vi "IT6322_Config_Link.vi"(8 "error in":errorcluster caption="错误输入（无错误）", 10 "等待时间(毫秒)":u32=100, 11 "MyIndex":u8) -> (0 "error out":errorcluster, 2 "返回值":string, 3 "状态":bool)   [LabVIEW 2015, in "IT6322.lvlib"]
uses:
  IT6322.lvlib
  <vilib>/Instr/_visa.llb/VISA Configure Serial Port (Instr).vi
panel:
  out "VISA":refnum<visa-resource-name>
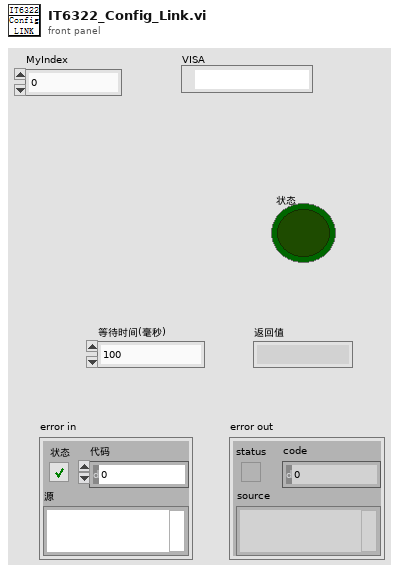
[diagram p1: front panel]
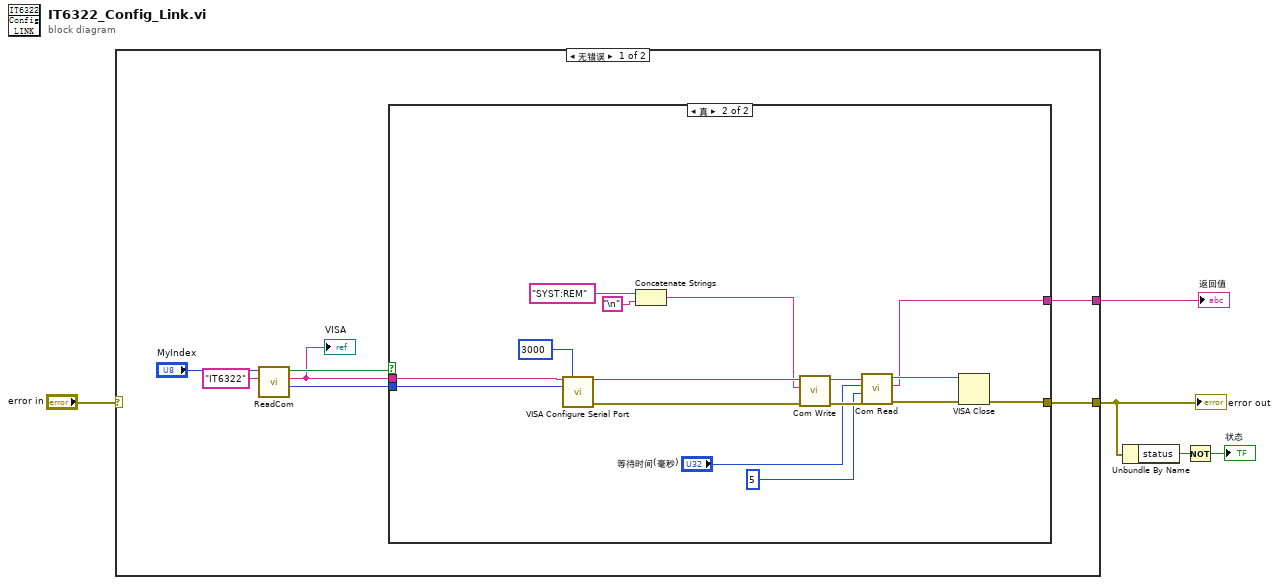
[diagram p0: block diagram]
diagram:
  n1 = case shown="无错误" "error in" {
    selector: "error in" -> [_ w29]
    tunnel: [w12 w29] -> w2
    tunnel: [w6 _] -> w3
    frame No Error {
      n2 = call "ReadCom.vi"("仪器名称"="IT6322", "MyIndex"="MyIndex") -> ("Baudrate"=w7:i32, "COM"=w8:string, "OK?"=w9:bool)  [unwired: 7 in]
      "VISA" <- w8
      n3 = case shown="真" w9 {
        tunnel: [_ w28] -> w12
        tunnel: w8 -> [_ w27]
        tunnel: w7 -> [_ w26]
        tunnel: [_ w18] -> w6
        frame False {
        }
        frame True {
          n4 = call-poly "VISA Configure Serial Port"("VISA resource name"=w27, "timeout (10sec)"=u32 3000, "baud rate (9600)"=w26) -> ("VISA resource name out"=w24:refnum<visa-resource-name>, "error out"=w23:errorcluster)  [unwired: 11 in]
          n5 = Concatenate Strings("SYST:REM", "\n") -> (w13:string)
          n6 = call "Com Write.vi"("错误输入（无错误）"=w23, "Wbuff"=w13, "VISA In"=w24) -> ("错误输出"=w21:errorcluster, "VISA Out"=w22:refnum<visa-resource-name>)  [unwired: 7 in]
          n7 = call "Com Read.vi"("错误输入（无错误）"=w21, "num"=u32 5, "超时"="等待时间(毫秒)", "VISA In"=w22) -> ("错误输出"=w20:errorcluster, "buff"=w18:string, "VISA Out"=w19:refnum<visa-resource-name>)  [unwired: 5 in]
          n8 = VISA Close(VISA resource name=w19, error in (no error)=w20) -> (error out=w28:errorcluster)
        }
      }
    }
    frame Error {
    }
  }
  "error out" <- w2
  "返回值" <- w3
  n9 = Unbundle By Name(w2) -> ("status"=w1:bool)
  n10 = Not(x=w1) -> (.not. x?=→"状态":bool)
